vi "06_Menu.vi"() -> ()   [LabVIEW 2020]
panel:
  in  "Button":bool
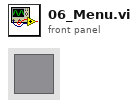
[diagram p1: front panel]
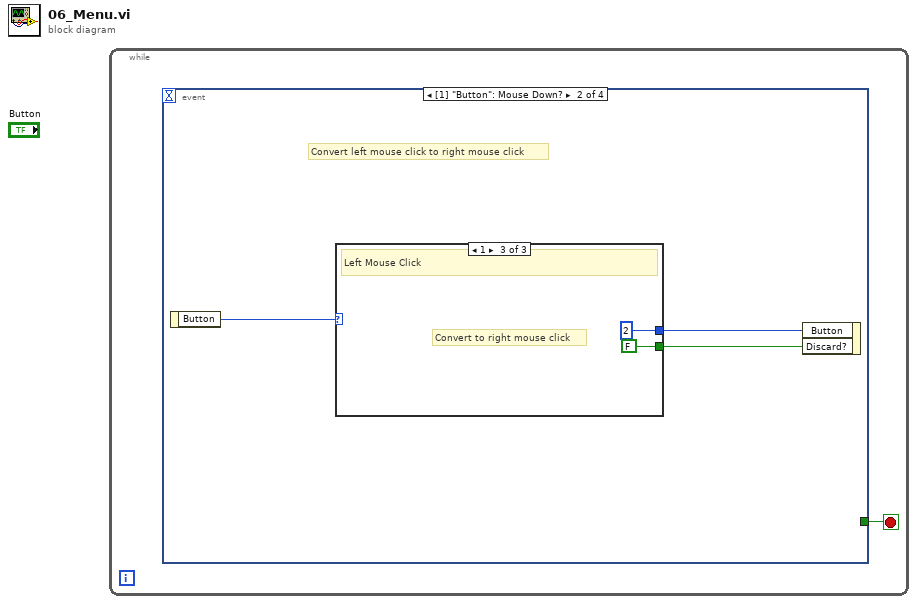
[diagram p0: block diagram]
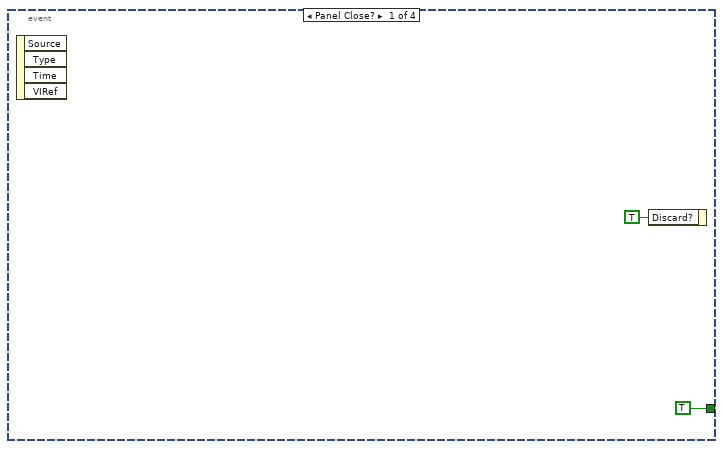
[diagram p2: hidden frame]
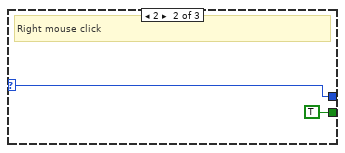
[diagram p4: hidden frame]
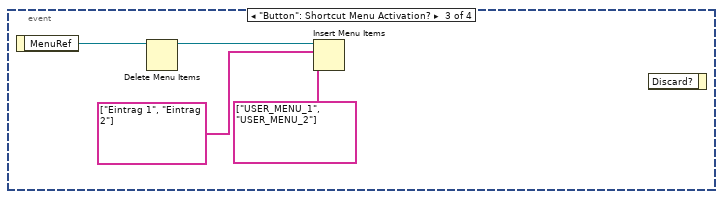
[diagram p5: hidden frame]
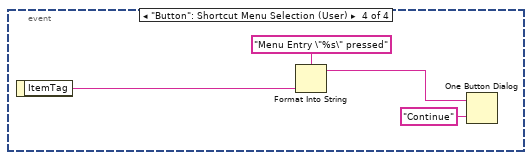
[diagram p6: hidden frame]
diagram:
  n1 = while {
    stop <- w1 stop-if-true
    n2 = event shown="[1] \"Button\": Mouse Down?" {
      selector: _ -> [_ _ _ _]
      dyn-events: _ -> [_ _ _ _]
      timeout: _ -> [_ _ _ _]
      tunnel: [TRUE _ _ _] -> w1
      event Panel Close? {
        n3 = event-data() -> ()  [unwired: 1 in, 4 out]
        n4 = event-data("Discard?"=TRUE) -> ()  [unwired: 1 in, 1 out]
      }
      event "Button": Mouse Down? {
        # "Convert left mouse click to right mouse click"
        n5 = event-data() -> ("Button"=w6:u16)  [unwired: 1 in]
        n6 = case shown="1" w6 {
          selector: w6 -> [w7 w9 _]
          tunnel: [w7 w9 u16 2 ("Button")] -> w5
          tunnel: [_ TRUE FALSE] -> w4
          frame Default {
          }
          frame 2 {
            # "Right mouse click"
          }
          frame 1 {
            # "Convert to right mouse click"
            # "Left Mouse Click"
          }
        }
        n7 = event-data("Button"=w5, "Discard?"=w4) -> ()  [unwired: 1 in, 1 out]
      }
      event "Button": Shortcut Menu Activation? {
        n8 = event-data() -> ("MenuRef"=w15:refnum<k9>)  [unwired: 1 in]
        n9 = Delete Menu Items(9:w15) -> (3:w14:refnum<k9>)  [unwired: 3 in, 1 out]
        n10 = Insert Menu Items(7:string[] ["USER_MENU_1", "USER_MENU_2"] ("item tags"), 8:string[] ["Eintrag 1", "Eintrag 2"] ("item names"), 9:w14) -> ()  [unwired: 3 in, 3 out]
        n11 = event-data() -> ()  [unwired: 2 in, 1 out]
      }
      event "Button": Shortcut Menu Selection (User) {
        n12 = event-data() -> ("ItemTag"=w18:string)  [unwired: 1 in]
        n13 = Format Into String(format string="Menu Entry \"%s\" pressed", w18) -> (resulting string=w17:string)  [unwired: 2 in, 1 out]
        n14 = One Button Dialog(message=w17, button name ("OK")="Continue") -> ()  [unwired: 1 out]
      }
    }
  }
